vi "eGateHSP_StartConfiguration.vi"(8 "Fehler (Eingang, kein Fehler)":errorcluster) -> (0 "Fehler (Ausgang)":errorcluster)   [LabVIEW 2016]
uses:
  eGateHighSpeedPort.dll
panel:
  out "Rückgabewert":i32
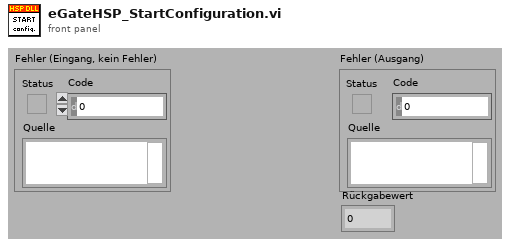
[diagram p1: front panel]
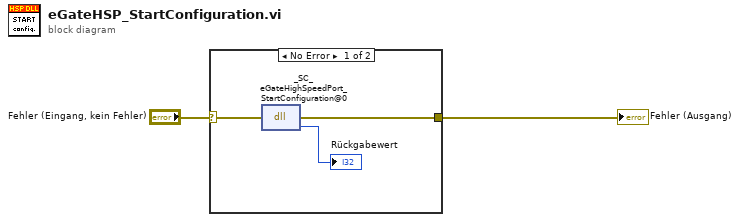
[diagram p0: block diagram]
diagram:
  n1 = case shown="No Error" "Fehler (Eingang, kein Fehler)" {
    selector: "Fehler (Eingang, kein Fehler)" -> [w5 _]
    tunnel: [w4 _] -> w1
    frame No Error {
      n2 = dll-call lib="eGateHighSpeedPort.dll" fn="_SC_eGateHighSpeedPort_StartConfiguration@0"(error in=w5) -> (error out=w4:errorcluster, "Rückgabewert"=→"Rückgabewert":i32)  [unwired: 2 in, 1 out]
    }
    frame Error {
    }
  }
  "Fehler (Ausgang)" <- w1
